vi "VI Tree.vi"   [LabVIEW 2022 SP3, in "LabVIEW-Config.lvlib"]
uses:
  LabVIEW-Config.lvlib
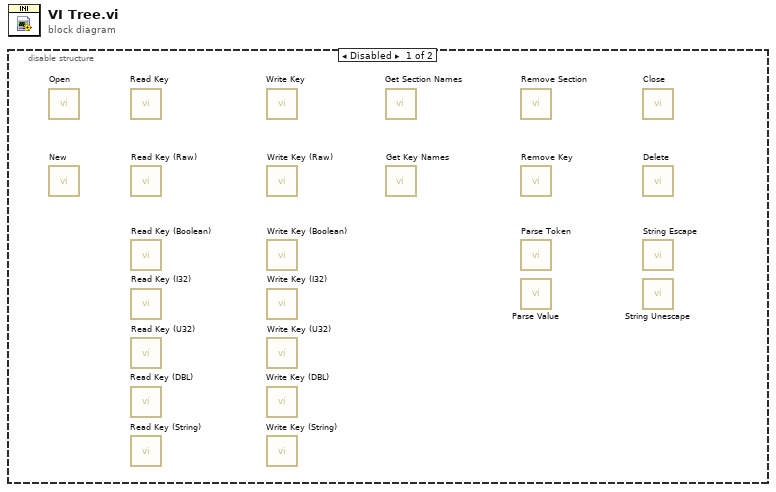
[diagram p0: block diagram]
diagram:
  n1 = disable-structure shown="Disabled" {
    frame Disabled {
      n2 = call "Open.vi"() -> ()  [unwired: 8 in, 4 out]
      n3 = call "New.vi"() -> ()  [unwired: 10 in, 2 out]
      n4 = call-poly "Read Key.vi"() -> ()  [unwired: 8 in, 4 out]
      n5 = call "Read Key (Raw).vi"() -> ()  [unwired: 8 in, 4 out]
      n6 = call "Read Key (Boolean).vi"() -> ()  [unwired: 8 in, 4 out]
      n7 = call "Read Key (I32).vi"() -> ()  [unwired: 8 in, 4 out]
      n8 = call "Read Key (U32).vi"() -> ()  [unwired: 8 in, 4 out]
      n9 = call "Read Key (DBL).vi"() -> ()  [unwired: 8 in, 4 out]
      n10 = call "Read Key (String).vi"() -> ()  [unwired: 8 in, 4 out]
      n11 = call-poly "Write Key.vi"() -> ()  [unwired: 9 in, 3 out]
      n12 = call "Write Key (Raw).vi"() -> ()  [unwired: 9 in, 3 out]
      n13 = call "Write Key (Boolean).vi"() -> ()  [unwired: 9 in, 3 out]
      n14 = call "Write Key (I32).vi"() -> ()  [unwired: 9 in, 3 out]
      n15 = call "Write Key (U32).vi"() -> ()  [unwired: 9 in, 3 out]
      n16 = call "Write Key (DBL).vi"() -> ()  [unwired: 9 in, 3 out]
      n17 = call "Write Key (String).vi"() -> ()  [unwired: 9 in, 3 out]
      n18 = call "Get Section Names.vi"() -> ()  [unwired: 9 in, 3 out]
      n19 = call "Get Key Names.vi"() -> ()  [unwired: 8 in, 4 out]
      n20 = call "Remove Section.vi"() -> ()  [unwired: 9 in, 3 out]
      n21 = call "Remove Key.vi"() -> ()  [unwired: 9 in, 3 out]
      n22 = call "Parse Token.vi"() -> ()  [unwired: 10 in, 2 out]
      n23 = call "Parse Value.vi"() -> ()  [unwired: 10 in, 2 out]
      n24 = call "Close.vi"() -> ()  [unwired: 10 in, 2 out]
      n25 = call "Delete.vi"() -> ()  [unwired: 8 in, 4 out]
      n26 = call "String Escape.vi"() -> ()  [unwired: 11 in, 1 out]
      n27 = call "String Unescape.vi"() -> ()  [unwired: 11 in, 1 out]
    }
    frame Enabled {
    }
  }
